vi "ToIOName.vi"(8 "error in":errorcluster, 11 "Generic":refnum<class "Generic.lvclass">) -> (0 "error out":errorcluster, 3 "IOName out":refnum<class "IOName.lvclass">)   [LabVIEW 2014, in "IOName.lvclass"]
uses:
  IOName.lvclass
  Generic/Generic.lvclass
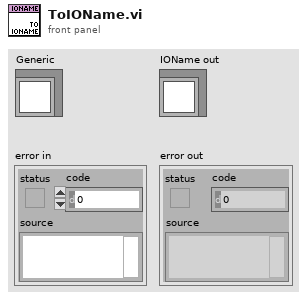
[diagram p1: front panel]
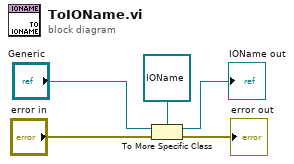
[diagram p0: block diagram]
diagram:
  n1 = To More Specific Class(target class=refnum<class "IOName.lvclass"> refnum ("Numeric in"), reference="Generic", error in="error in") -> (specific class reference=→"IOName out":refnum<class "IOName.lvclass">, error out=→"error out":errorcluster)
